vi "Semaforo.vi"() -> ()   [LabVIEW 2018]
panel:
  out "TEMPO":i32
  in  "stop":bool
  in  "Cross Button":bool
  out "Red Light":bool
  out "Yellow Light":bool
  out "Green Light":bool
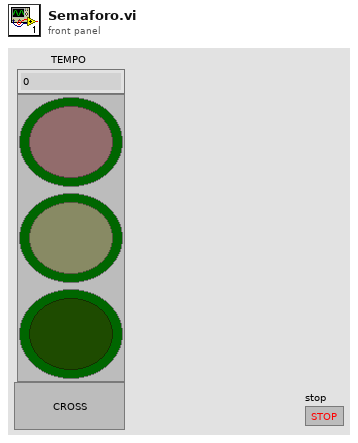
[diagram p1: front panel]
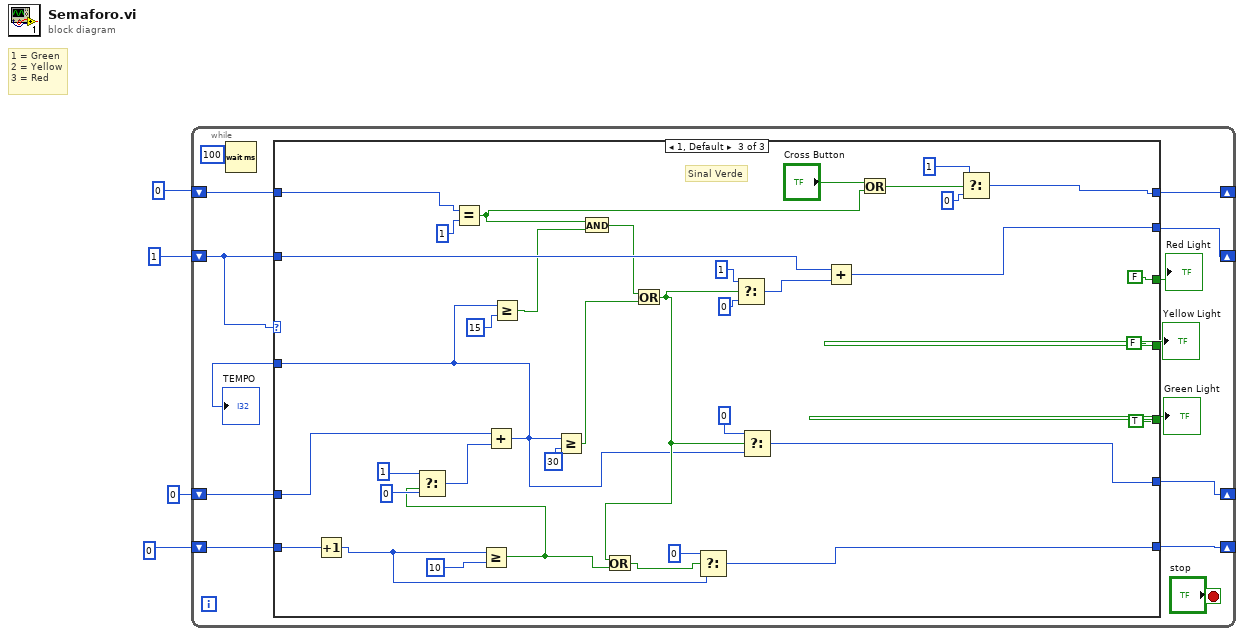
[diagram p0: block diagram]
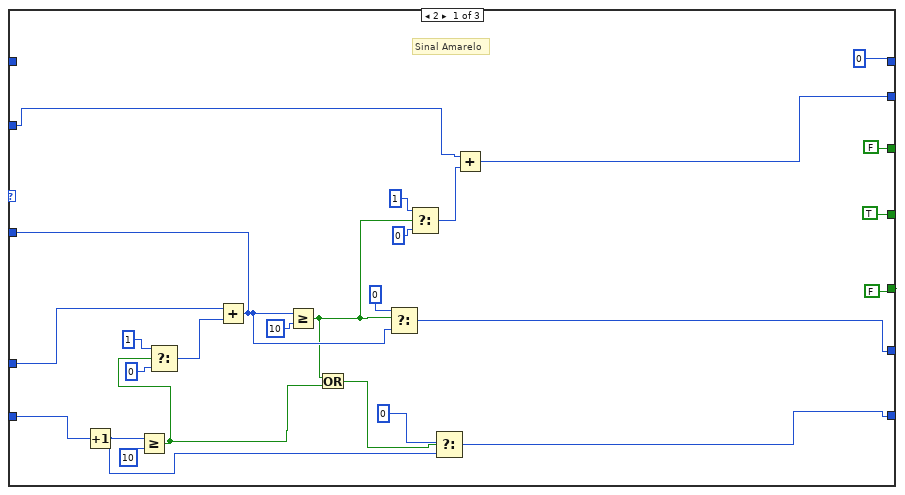
[diagram p2: hidden frame]
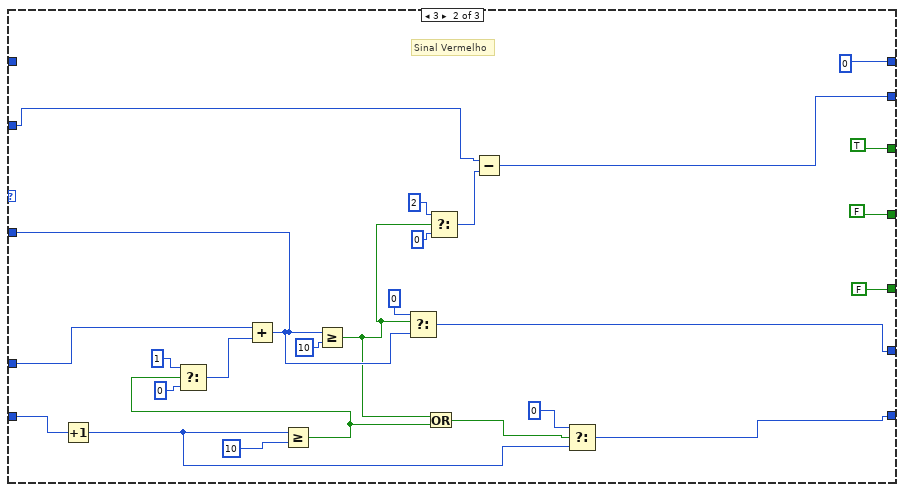
[diagram p3: hidden frame]
diagram:
  # "1 = Green\n2 = Yellow\n3 = Red"
  n1 = while {
    shift-right: [w12] -> _
    shift-left: 0 -> [w13]
    shift-right: [w7] -> _
    shift-left: 1 -> [w8]
    shift-right: [w9] -> _
    shift-left: 0 -> [w11]
    shift-right: [w6] -> _
    shift-left: 0 -> [w5]
    stop <- "stop" stop-if-true
    n2 = Wait (ms)(milliseconds to wait=u32 100) -> ()  [unwired: 1 out]
    n3 = case shown="1, Default" w8 {
      tunnel: [FALSE FALSE TRUE] -> w18
      tunnel: [TRUE FALSE FALSE] -> w17
      tunnel: [FALSE TRUE FALSE] -> w16
      tunnel: w13 -> [w38 w63 w99]
      tunnel: [w23 w49 w85] -> w12
      tunnel: w11 -> [w33 w60 w94]
      tunnel: [w28 w53 w74] -> w10
      tunnel: [w25 w52 w92] -> w9
      tunnel: w8 -> [w27 w51 w88]
      tunnel: [w26 w50 w87] -> w7
      tunnel: [0 0 w78] -> w6
      tunnel: w5 -> [_ _ w76]
      frame 2 {
        # "Sinal Amarelo"
        n4 = Increment(x=w38) -> (x+1=w24:i32)
        n5 = Greater Or Equal?(x=w24, y=10) -> (x >= y?=w21:bool)
        n6 = Select(t=1, s=w21, f=0) -> (s? t:f=w37:i32)
        n7 = Add(x=w33, y=w37) -> (x+y=w28:i32)
        n8 = Greater Or Equal?(x=w28, y=10) -> (x >= y?=w22:bool)
        n9 = Or(x=w22, y=w21) -> (x .or. y?=w20:bool)
        n10 = Select(t=0, s=w22, f=w28) -> (s? t:f=w25:i32)
        n11 = Select(t=1, s=w22, f=0) -> (s? t:f=w32:i32)
        n12 = Select(t=0, s=w20, f=w24) -> (s? t:f=w23:i32)
        n13 = Add(x=w27, y=w32) -> (x+y=w26:i32)
      }
      frame 3 {
        # "Sinal Vermelho"
        n14 = Increment(x=w63) -> (x+1=w48:i32)
        n15 = Greater Or Equal?(x=w48, y=10) -> (x >= y?=w46:bool)
        n16 = Select(t=1, s=w46, f=0) -> (s? t:f=w59:i32)
        n17 = Add(x=w60, y=w59) -> (x+y=w53:i32)
        n18 = Greater Or Equal?(x=w53, y=10) -> (x >= y?=w47:bool)
        n19 = Select(t=0, s=w47, f=w53) -> (s? t:f=w52:i32)
        n20 = Or(x=w47, y=w46) -> (x .or. y?=w45:bool)
        n21 = Select(t=2, s=w47, f=0) -> (s? t:f=w57:i32)
        n22 = Subtract(x=w51, y=w57) -> (x-y=w50:i32)
        n23 = Select(t=0, s=w45, f=w48) -> (s? t:f=w49:i32)
      }
      frame 1, Default {
        # "Sinal Verde"
        n24 = Increment(x=w99) -> (x+1=w84:i32)
        n25 = Equal?(x=w76, y=1) -> (x = y?=w69:bool)
        n26 = Greater Or Equal?(x=w84, y=10) -> (x >= y?=w83:bool)
        n27 = Select(t=1, s=w83, f=0) -> (s? t:f=w98:i32)
        n28 = Add(x=w94, y=w98) -> (x+y=w74:i32)
        n29 = Greater Or Equal?(x=w74, y=15) -> (x >= y?=w73:bool)
        n30 = Greater Or Equal?(x=w74, y=30) -> (x >= y?=w86:bool)
        n31 = And(x=w69, y=w73) -> (x .and. y?=w72:bool)
        n32 = Or(x=w72, y=w86) -> (x .or. y?=w81:bool)
        n33 = Or(x=w81, y=w83) -> (x .or. y?=w82:bool)
        n34 = Select(t=0, s=w82, f=w84) -> (s? t:f=w85:i32)
        n35 = Select(t=1, s=w81, f=0) -> (s? t:f=w89:i32)
        n36 = Select(t=0, s=w81, f=w74) -> (s? t:f=w92:i32)
        n37 = Add(x=w88, y=w89) -> (x+y=w87:i32)
        n38 = Or(x="Cross Button", y=w69) -> (x .or. y?=w71:bool)
        n39 = Select(t=1, s=w71, f=0) -> (s? t:f=w78:i32)
      }
    }
    "Green Light" <- w18
    "Yellow Light" <- w17
    "Red Light" <- w16
    "TEMPO" <- w10
  }
